vi "Handle Messages.vi"(8 "error in (no error)":errorcluster, 9 "Message Data":variant, 10 "Message":string, 11 "Demo Process In":refnum<class "Demo Process.lvclass">) -> (0 "error out":errorcluster, 3 "Demo Process Out":refnum<class "Demo Process.lvclass">)   [LabVIEW 2020, in "Test.lvlib" / "Demo Process.lvclass"]
uses:
  Demo Process.lvclass
  <vilib>/Astemes/Triarc Framework/Process/Process.lvclass
  Demo Process.lvclass/Demo Process.ctl
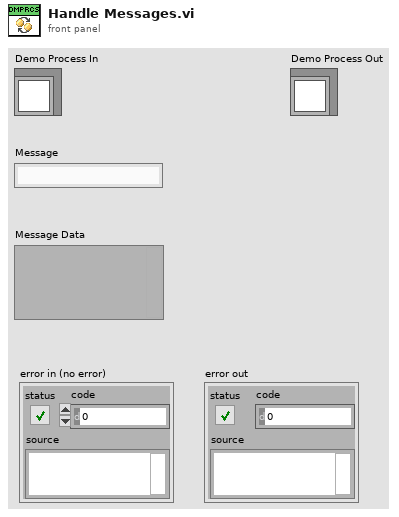
[diagram p1: front panel]
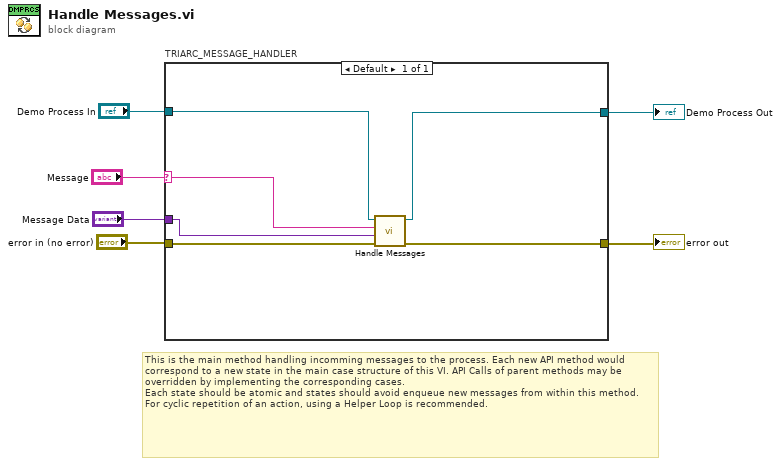
[diagram p0: block diagram]
diagram:
  # "This is the main method handling incomming messages to the process. Each new API method would correspond to a new state in the main case structure of this VI. API Calls of parent methods may be overridden by implementing the corresponding cases.\nEach state should be atomic and states should avoid enqueue new messages from within this method. For cyclic repetition of an action, using a Helper Loop is recommended."
  n1 = case "TRIARC_MESSAGE_HANDLER" shown="Default" "Message" {
    selector: "Message" -> [w10]
    tunnel: "error in (no error)" -> [w9]
    tunnel: "Demo Process In" -> [w12]
    tunnel: "Message Data" -> [w11]
    tunnel: [w8] -> w2
    tunnel: [w7] -> w1
    frame Default {
      n2 = call-parent "Handle Messages.vi"("error in (no error)"=w9, "Message Data"=w11, "Message"=w10, "Process In"=w12) -> ("error out"=w8:errorcluster, "Process Out"=w7:refnum<class "Demo Process.lvclass">)  [unwired: 6 in]
    }
  }
  "error out" <- w2
  "Demo Process Out" <- w1
